vi "Format&SaveDataClean.vi"(0 "Data_Angle_deg":sgl[](array[numeric])=[490.08, 490.12, 490.16, 490.2], 1 "Data_PLInt_cts":i32[](array[numeric])=[1, 3, 2, 1], 3 "Data_FSMPos_V":dbl[][](array[numeric]), 4 "Data_CCD_px":dbl[][](array[numeric]), 5 "Measurement type":T3(ring)=enum."Contrast", 6 "L2Exc_deg":dbl[](array[numeric]), 7 "Suppl_2D":dbl[][](array[numeric]), 8 "L2Det_deg":dbl[](array[numeric]), 9 "Params Save":T2, 12 "Main 3D Data to write":dbl[][][](array[numeric])=[[[2.2, 4.4, 3.3, 5.5, 6.6]]], 13 "Suppl":dbl[](array[numeric]), 15 "Suppl_3D":dbl[][][](array[numeric])) -> (10 "WrittenDatasetName":string, 14 "Log File Out":string)   [LabVIEW 2019]
uses:
  TypeDefs/AcqMode.ctl
  <vilib>/UPVI/lvhdf5/dataset.llb/LVH5D Operation.ctl
  <vilib>/Utility/miscctls.llb/LVRectTypeDef.ctl
  <vilib>/UPVI/lvhdf5/attribute.llb/LVH5A Operation.ctl
  <vilib>/UPVI/lvhdf5/group.llb/H5G_obj_t.ctl
  <vilib>/UPVI/lvhdf5/identifier.llb/Not an HDF5 Refnum Constant.vi
  <vilib>/UPVI/lvhdf5/common.llb/To HDF5 Ref.vi
  <vilib>/UPVI/lvhdf5/group.llb/OpenCreateGroup (String).vi
  <vilib>/Utility/VariantDataType/GetClusterInfo.vi
  <vilib>/Utility/VariantDataType/GetTypeInfo.vi
  <vilib>/UPVI/lvhdf5/utility.llb/Select HDF5 Dialog.vi
  <vilib>/UPVI/lvhdf5/utility.llb/Select HDF5 Dialog (Object Only).vi
  <vilib>/UPVI/lvhdf5/dataset.llb/Simple H5Dwrite (Variant).vi
  <vilib>/UPVI/lvhdf5/attribute.llb/Write Multiple Attributes.vi
  <vilib>/UPVI/lvhdf5/dataset.llb/H5Dclose.vi
  <vilib>/UPVI/lvhdf5/dataset.llb/Write Dataset with Attributes.xnode
  <vilib>/UPVI/lvhdf5/library.llb/HDF5 Ref.ctl
  <vilib>/UPVI/lvhdf5/attribute.llb/Cluster to Attribute Array.xnode
  <vilib>/Utility/error.llb/Error Cluster From Error Code.vi
  <vilib>/UPVI/lvhdf5/dataset.llb/OpenCreateReplace Dataset by Element Type.vi
  <vilib>/UPVI/lvhdf5/dataspace.llb/H5Sselect_hyperslab.vi
  <vilib>/UPVI/lvhdf5/dataset.llb/H5Dwrite (Variant).vi
  <vilib>/UPVI/lvhdf5/dataset.llb/H5Dget_space.vi
  <vilib>/UPVI/lvhdf5/attribute.llb/private/LVH5AwriteWDTAttrs.vi
  <vilib>/UPVI/lvhdf5/dataspace.llb/H5Sclose.vi
  <vilib>/UPVI/lvhdf5/file.llb/LVH5F Operation.ctl
  <vilib>/UPVI/lvhdf5/utility.llb/Select HDF5 Dialog (File and Object).vi
  <vilib>/Utility/VariantDataType/VariantType.lvlib
panel:
  in  "ESource":enum16{"P", "CW", "SK"}(ring)
  in  "Acq Mode":T1=enum."Spectrum" caption="Acq mode"
  in  "Log File In":string
  out "File path":path=path "Cluster Attributes.hdf5"
  in  "DatasetName":string="test"
  in  "Main 2D Data to write":dbl[][](array[numeric])=[[2.2, 4.4, 3.3, 5.5, 6.6]]
  in  "Comment":string="This is a test"
  out "Date":string="2006-1-11"
  in  "T_K":dbl=5.0
  in  "EPow_uW":dbl=0.21
  in  "EWL_nm":dbl=450.0
  in  "Time_ms":dbl=500.0
  in  "Det_Mono1_EntSlit_mm":dbl=0.01
  in  "Det_Mono1_ExtSlit_mm":dbl=0.01
  in  "WL_nm":sgl[](array[numeric])=[490.08, 490.12, 490.16, 490.2]
  in  "MeasurementName":string
  in  "FileName":string="test"
  in  "Det_Mono1_CenterWL_nm":dbl=490.0
  out "Exists":bool
  out "Homonyms":string[](array[string])
  out "size(s)":i32
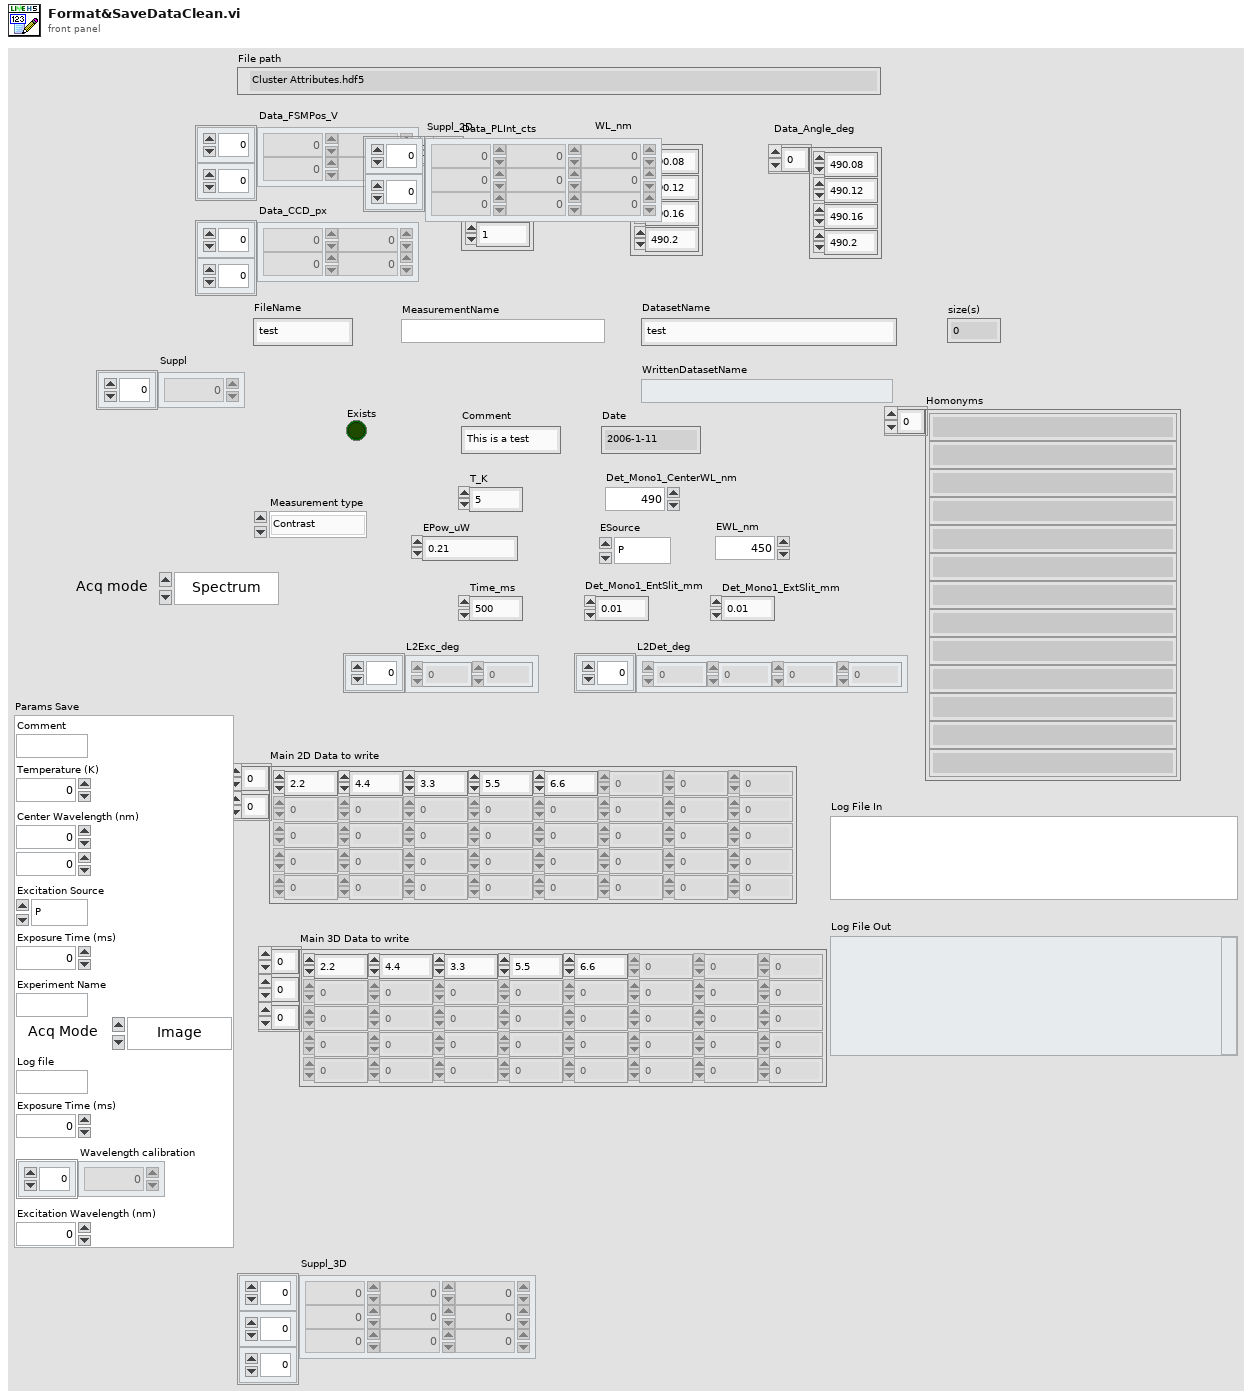
[diagram p1: front panel]
types:
  T1 = typedef "AcqMode.ctl" = enum16{"Image", "Spectrum", "APD 1", "APD 2", "APD 1+2"}
  T2 = cluster{"Comment":string, "Temperature (K)":dbl, "Center Wavelength (nm)":dbl, "Numeric":dbl, "Excitation Source":enum16{"P", "CW", "SK"}, "Exposure Time (ms)":dbl, "Experiment Name":string, "Acq Mode":T1, "Log file":string, "Exposure Time (ms)":dbl, "Wavelength calibration":dbl[], "Excitation Wavelength (nm)":dbl}
  T3 = enum16{"Time Trace", "Contrast", "XY Intensity Map", "Polarisation", "Spectrum", "Michelson"}
  T4 = typedef "LVH5D Operation.ctl" = enum16{"open", "replace", "create", "open or create", "create or replace", "create or replace with confirmation"}
  T5 = typedef "LVH5A Operation.ctl" = enum16{"open", "replace", "create", "open or create", "create or replace", "create or replace with confirmation"}
  T6 = typedef "LVRectTypeDef.ctl" = cluster{"Left":i16, "Top":i16, "Right":i16, "Bottom":i16}
  T7 = cluster{"Behavior":enum32{"Invalid", "Default", "Floating", "Floating/Auto-Hide", "Modal"}, "Position":T6, "Center":bool, "Title":string}
  T8 = typedef "LVH5F Operation.ctl" = enum16{"open", "open or create", "create or replace", "create or replace (with confirmation)", "create", "open (read only)"}
  T9 = typedef "H5G_obj_t.ctl" = i32
  T10 = cluster{"Object Types (any)":T9[], "Object Pattern":string}
  T11 = typedef "HDF5 Ref.ctl" = refnum<k1>
  T12 = cluster{"date/time string":string, "Comment":string, "T_K":dbl, "ESource":enum16{"P", "CW", "SK"}, "EWL_nm":dbl, "EPow_uW":dbl, "Time_ms":dbl, "WL_nm":sgl[], "Suppl":dbl[], "L2Exc_deg":dbl[], "L2Det_deg":dbl[]}
  T13 = cluster{"date/time string":string, "Comment":string, "T_K":dbl, "ESource":enum16{"P", "CW", "SK"}, "EWL_nm":dbl, "EPow_uW":dbl, "Time_ms":dbl, "WL_nm":sgl[], "Suppl_2D":dbl[][], "L2Exc_deg":dbl[], "L2Det_deg":dbl[]}
  T14 = cluster{"date/time string":string, "Comment":string, "T_K":dbl, "ESource":enum16{"P", "CW", "SK"}, "EWL_nm":dbl, "EPow_uW":dbl, "Time_ms":dbl, "WL_nm":sgl[], "Suppl_3D":dbl[][][], "L2Exc_deg":dbl[], "L2Det_deg":dbl[]}
  T15 = cluster{"date/time string":string, "Comment":string, "T_K":dbl, "ESource":enum16{"P", "CW", "SK"}, "EWL_nm":dbl, "EPow_uW":dbl, "Time_ms":dbl, "WL_nm":sgl[], "Suppl":dbl[], "L2Exc_deg":dbl[], "L2Det_deg":dbl[], "WL_nm":sgl[]}
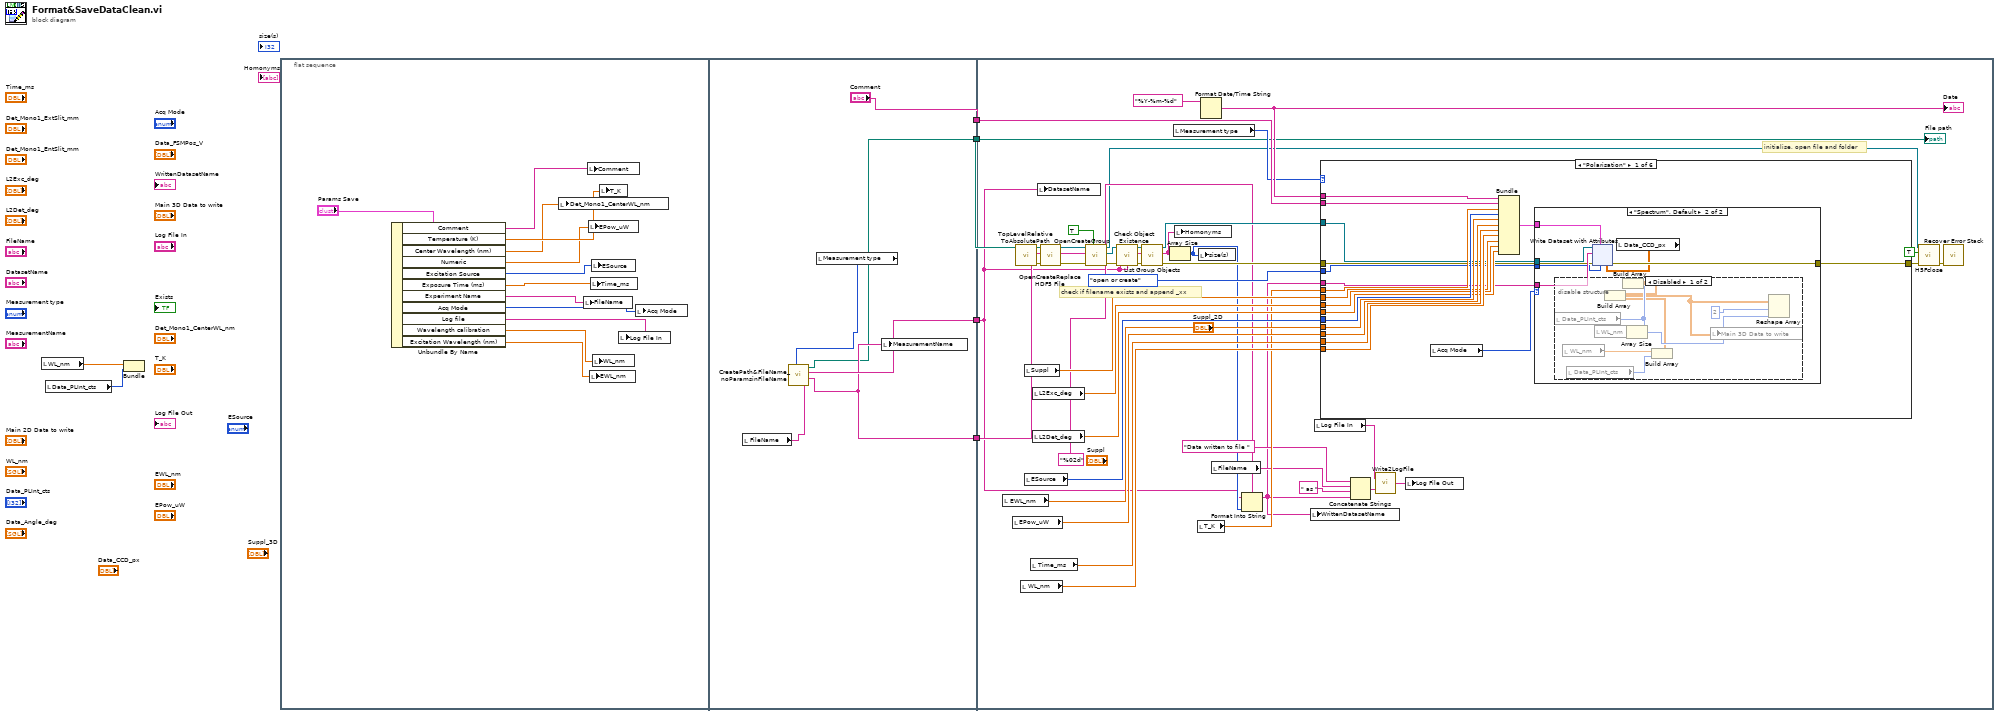
[diagram p0: block diagram]
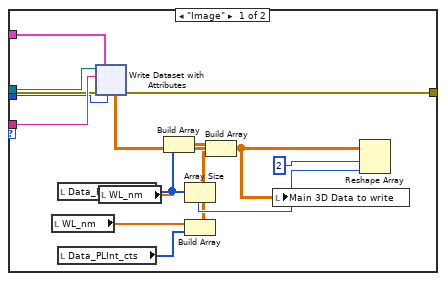
[diagram p2: hidden frame]
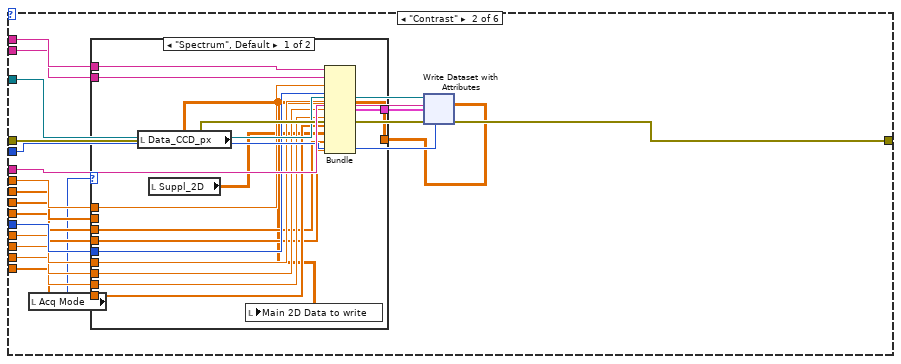
[diagram p4: hidden frame]
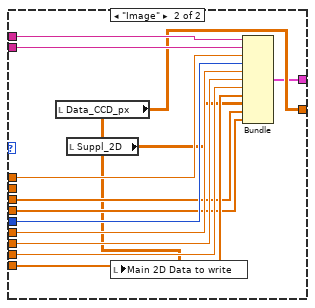
[diagram p5: hidden frame]
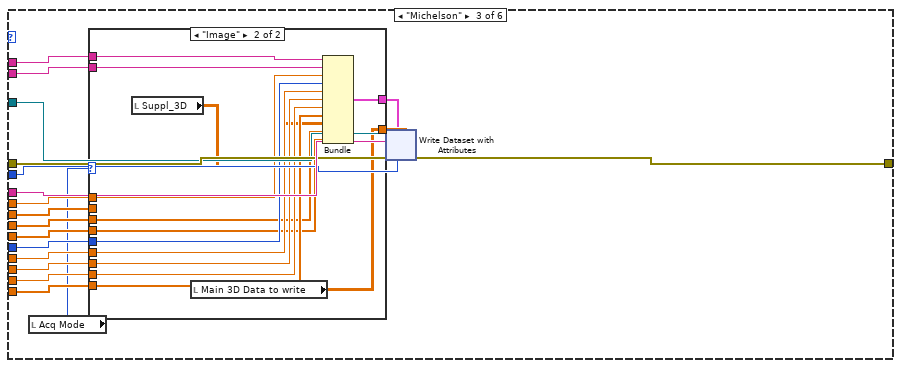
[diagram p6: hidden frame]
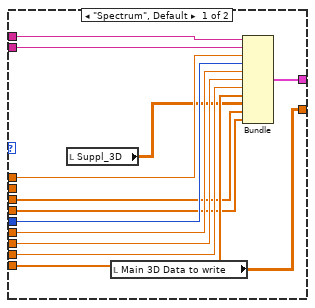
[diagram p7: hidden frame]
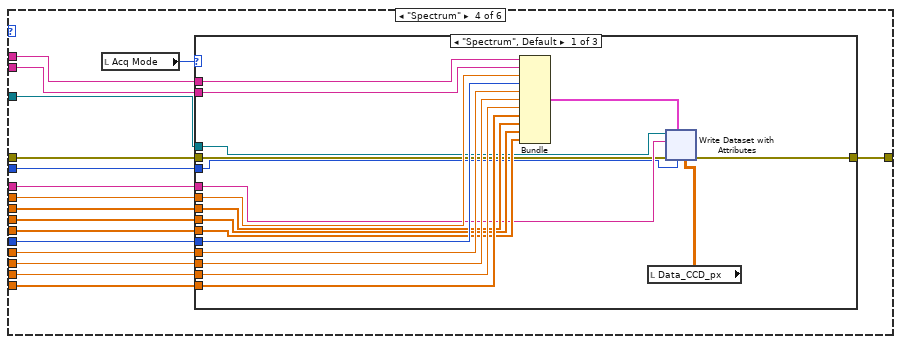
[diagram p8: hidden frame]
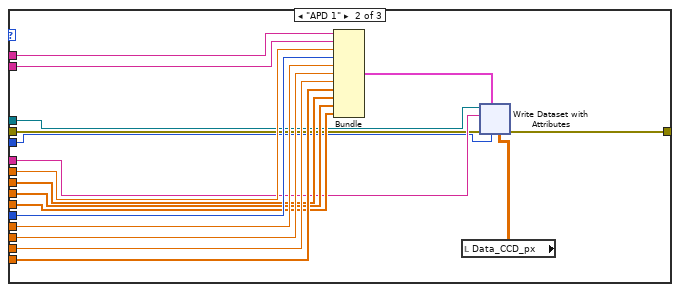
[diagram p9: hidden frame]
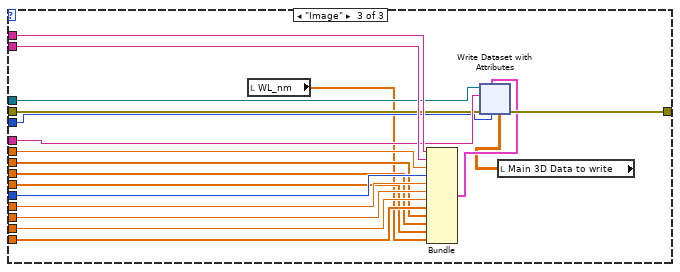
[diagram p10: hidden frame]
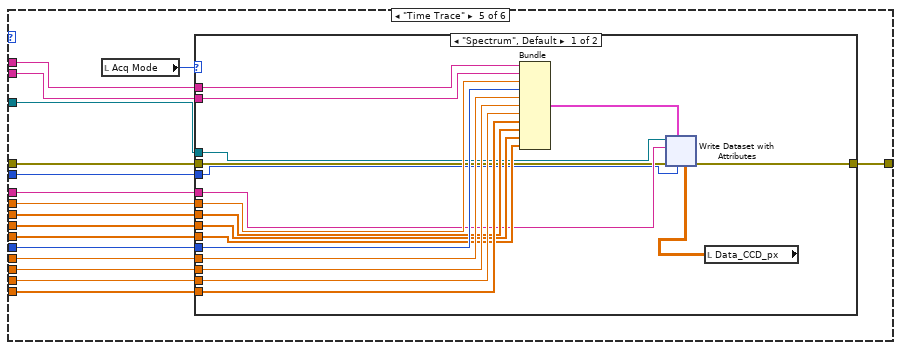
[diagram p11: hidden frame]
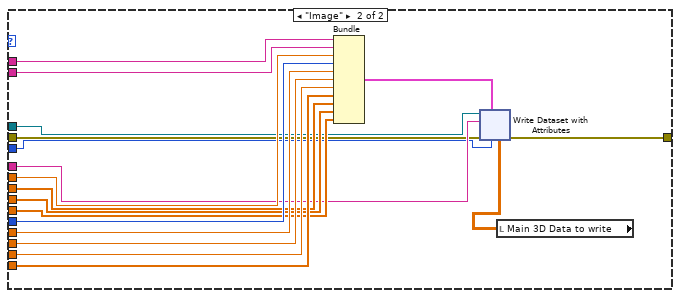
[diagram p12: hidden frame]
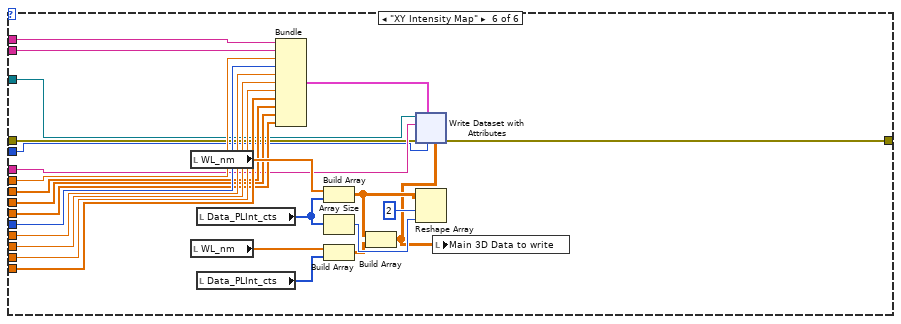
[diagram p13: hidden frame]
diagram:
  n1 = local read "WL_nm"() -> (w5:sgl[])
  n2 = local read "Data_PLInt_cts"() -> (w6:i32[])
  n3 = Bundle("WL_nm"=w5, "Data_PLInt_cts"=w6) -> ()  [unwired: 1 in, 1 out]
  n4 = flat-sequence {
    tunnel: ["Comment"] -> w4
    tunnel: [w22] -> w3
    tunnel: [w21] -> w2
    tunnel: [w20] -> w1
    tunnel: w4 -> [w53]
    tunnel: w3 -> [w25]
    tunnel: w2 -> [w43]
    tunnel: w1 -> [w36]
    frame #0 {
      n5 = Unbundle By Name("Params Save") -> ("Comment"=w17:string, "Temperature (K)"=w16:dbl, "Center Wavelength (nm)"=w14:dbl, "Numeric"=w15:dbl, "Excitation Source"=w13:enum16{"P", "CW", "SK"}, "Exposure Time (ms)"=w12:dbl, "Experiment Name"=w9:string, "Acq Mode"=w10:T1, "Log file"=w11:string, "Wavelength calibration"=w7:dbl[], "Excitation Wavelength (nm)"=w8:dbl)
      n6 = local write "Det_Mono1_CenterWL_nm"(w14) -> ()
      n7 = local write "FileName"(w9) -> ()
      n8 = local write "Comment"(w17) -> ()
      n9 = local write "EPow_uW"(w15) -> ()
      n10 = local write "EWL_nm"(w8) -> ()
      n11 = local write "Time_ms"(w12) -> ()
      n12 = local write "ESource"(w13) -> ()
      n13 = local write "WL_nm"(w7) -> ()
      n14 = local write "T_K"(w16) -> ()
      n15 = local write "Log File In"(w11) -> ()
      n16 = local write "Acq Mode"(w10) -> ()
    }
    frame #1 {
      n17 = local read "FileName"() -> (w19:string)
      n18 = local read "Measurement type"() -> (w23:T3)
      n19 = call "CreatePath&FileName_noParamsinFileName.vi"("FileName"=w19, "Measurement type"=w23) -> ("MeasurementGroupName"=w21:string, "DatasetName"=w22:string, "File path"=w20:path)  [unwired: 4 in]
      n20 = local write "MeasurementName"(w21) -> ()
    }
    frame #2 {
      # "initialise, open file and folder"
      # "check if filename exists and append _xx"
      n21 = local read "EWL_nm"() -> (w56:dbl)
      n22 = local read "EPow_uW"() -> (w57:dbl)
      n23 = call "TopLevelRelativeToAbsolutePath.vi"("Path Relative to Top Level VI"=w36) -> ("error out"=w34:errorcluster, "Absolute path"=w33:path)  [unwired: 9 in]
      n24 = local read "WL_nm"() -> (w59:sgl[])
      n25 = local read "Suppl"() -> (w60:dbl[])
      n26 = local read "ESource"() -> (w55:enum16{"P", "CW", "SK"})
      n27 = local read "Time_ms"() -> (w58:dbl)
      n28 = local read "L2Exc_deg"() -> (w61:dbl[])
      n29 = local read "L2Det_deg"() -> (w62:dbl[])
      n30 = local write "DatasetName"(w25) -> ()
      n31 = call <vilib>:"OpenCreateReplace HDF5 File.vi"("error in (no error)"=w34, "path"=w33) -> ("error out"=w38:errorcluster, "HDF5 Ref out"=w37:T11)  [unwired: 6 in]
      n32 = call-poly <vilib>:"OpenCreateGroup.vi"("Create if not found (F)"=TRUE, "error in (no error)"=w38, "Group"=w43, "HDF5 Ref"=w37) -> ("error out"=w46:errorcluster, "HDF5 Group Ref"=w45:T11, "HDF5 Ref out"=w41:T11)  [unwired: 5 in]
      n33 = call <vilib>:"Check Object Existence.vi"("error in (no error)"=w46, "name"=w25, "HDF5 Ref"=w45) -> ("error out"=w47:errorcluster, "HDF5 Ref out"=w48:T11)  [unwired: 4 in, 1 out]
      n34 = call <vilib>:"List Group Objects.vi"("error in (no error)"=w47, "pattern"=w25, "HDF5 Loc Ref"=w48) -> ("error out"=w63:errorcluster, "Object Names"=w49:string[], "HDF5 Loc Ref out"=w65:T11)  [unwired: 3 in, 1 out]
      n35 = Array Size(array=w49) -> (size(s)=w50:i32)
      n36 = local read "Measurement type"() -> (w42:T3)
      n37 = local write "Homonyms"(w49) -> ()
      n38 = local read "T_K"() -> (w54:dbl)
      n39 = local write "size(s)"(w50) -> ()
      n40 = Format Date/Time String(time format string (%c)="%Y-%m-%d") -> (date/time string=w52:string)  [unwired: 2 in]
      "Date" <- w52
      n41 = local read "FileName"() -> (w31:string)
      n42 = Format Into String(format string="%02d", initial string=w25, w50) -> (resulting string=w29:string)  [unwired: 1 in, 1 out]
      n43 = local write "WrittenDatasetName"(w29) -> ()
      n44 = local read "Log File In"() -> (w28:string)
      n45 = case shown="\"Polarisation\"" w42 {
        tunnel: w52 -> [w84 w762 w1121 w1478 w2494 w3180]
        tunnel: w53 -> [w83 w761 w1120 w1477 w2493 w3179]
        tunnel: w54 -> [w82 w760 w1119 w1476 w2492 w3178]
        tunnel: w55 -> [w81 w759 w1118 w1475 w2491 w3177]
        tunnel: w56 -> [w80 w758 w1117 w1474 w2490 w3176]
        tunnel: w57 -> [w79 w757 w1116 w1473 w2489 w3175]
        tunnel: w58 -> [w78 w756 w1115 w1472 w2488 w3174]
        tunnel: w59 -> [w77 w755 w1114 w1471 w2487 w3173]
        tunnel: w60 -> [w76 w754 w1113 w1470 w2486 w3172]
        tunnel: w61 -> [w75 w753 w1112 w1469 w2485 w3171]
        tunnel: w62 -> [w74 w752 w1111 w1468 w2484 w3170]
        tunnel: w29 -> [w73 w751 w1110 w1467 w2483 w3169]
        tunnel: w63 -> [w72 w750 w1109 w1466 w2482 w3168]
        tunnel: LVH5D_Operation."open or create" ("operation (open or create)") -> [w71 w749 w1108 w1465 w2481 w3167]
        tunnel: w65 -> [w70 w748 w1107 w1464 w2480 w3166]
        tunnel: [w69 w747 w1106 w1463 w2479 w3165] -> w66
        frame "Polarisation" {
          n46 = local read "Acq Mode"() -> (w68:T1)
          n47 = Bundle("date/time string"=w84, "Comment"=w83, "T_K"=w82, "ESource"=w81, "EWL_nm"=w80, "EPow_uW"=w79, "Time_ms"=w78, "WL_nm"=w77, "Suppl"=w76, "L2Exc_deg"=w75, "L2Det_deg"=w74) -> (w67:T12)  [unwired: 1 in]
          n48 = case shown="\"Spectrum\", Default" w68 {
            tunnel: w73 -> [w95 w420]
            tunnel: w72 -> [w94 w419]
            tunnel: w71 -> [w93 w418]
            tunnel: w70 -> [w92 w417]
            tunnel: [w91 w416] -> w69
            tunnel: w67 -> [w85 w415]
            frame "Image" {
              n49 = local read "WL_nm"() -> (w90:sgl[])
              n50 = local read "Data_PLInt_cts"() -> (w97:i32[])
              n51 = local read "Data_PLInt_cts"() -> (w89:i32[])
              n52 = local read "WL_nm"() -> (w96:sgl[])
              n53 = Build Array(w96, w97) -> (w87:sgl[][])
              n54 = Array Size(array=w97) -> (size(s)=w98:i32)
              n55 = Build Array(w90, w89) -> (w88:sgl[][])
              n56 = Build Array(w87, w88) -> (w86:sgl[][][])
              n57 = xnode "Write Dataset with Attributes"("Dataset Path"=w95, "error in (no error)"=w94, "operation (open or create)"=w93, "HDF5 Path or Ref"=w92, "Attribute Value(s)"=w85, "Data"=w86) -> ("error out"=w91:errorcluster)  [unwired: 2 in, 2 out]
              n58 = local write "Main 3D Data to write"(w86) -> ()
              n59 = Reshape Array(w86, 2 ("dimension size"), w98) -> ()  [unwired: 1 out]
            }
            frame "Spectrum", Default {
              n60 = disable-structure shown="Disabled" {
                frame Disabled {
                  n61 = local read "Data_PLInt_cts"() -> (w427:i32[])
                  n62 = local read "WL_nm"() -> (w425:sgl[])
                  n63 = local read "Data_PLInt_cts"() -> (w424:i32[])
                  n64 = local read "WL_nm"() -> (w426:sgl[])
                  n65 = Build Array(w426, w427) -> (w422:sgl[][])
                  n66 = Array Size(array=w427) -> (size(s)=w428:i32)
                  n67 = Build Array(w425, w424) -> (w423:sgl[][])
                  n68 = Build Array(w422, w423) -> (w421:sgl[][][])
                  n69 = local write "Main 3D Data to write"(w421) -> ()
                  n70 = Reshape Array(w421, 2 ("dimension size"), w428) -> ()  [unwired: 1 out]
                }
                frame Enabled {
                }
              }
              n71 = local read "Data_CCD_px"() -> (w414:dbl[][])
              n72 = xnode "Write Dataset with Attributes"("Dataset Path"=w420, "error in (no error)"=w419, "operation (open or create)"=w418, "HDF5 Path or Ref"=w417, "Attribute Value(s)"=w415, "Data"=w414) -> ("error out"=w416:errorcluster)  [unwired: 2 in, 2 out]
            }
          }
        }
        frame "Contrast" {
          n73 = local read "Acq Mode"() -> (w745:T1)
          n74 = case shown="\"Spectrum\", Default" w745 {
            tunnel: w762 -> [w775 w788]
            tunnel: w761 -> [w774 w787]
            tunnel: w760 -> [w773 w786]
            tunnel: w759 -> [w772 w785]
            tunnel: w758 -> [w771 w784]
            tunnel: w757 -> [w770 w783]
            tunnel: w756 -> [w769 w782]
            tunnel: w755 -> [w768 w781]
            tunnel: w754 -> [_ _]
            tunnel: w753 -> [w767 w780]
            tunnel: w752 -> [w766 w779]
            tunnel: [w765 w778] -> w746
            tunnel: [w763 w777] -> w744
            frame "Spectrum", Default {
              n75 = local read "Data_CCD_px"() -> (w765:dbl[][])
              n76 = local read "Suppl_2D"() -> (w764:dbl[][])
              n77 = local write "Main 2D Data to write"(w765) -> ()
              n78 = Bundle("date/time string"=w775, "Comment"=w774, "T_K"=w773, "ESource"=w772, "EWL_nm"=w771, "EPow_uW"=w770, "Time_ms"=w769, "WL_nm"=w768, "Suppl_2D"=w764, "L2Exc_deg"=w767, "L2Det_deg"=w766) -> (w763:T13)  [unwired: 1 in]
            }
            frame "Image" {
              n79 = local read "Data_CCD_px"() -> (w778:dbl[][])
              n80 = local read "Suppl_2D"() -> (w776:dbl[][])
              n81 = local write "Main 2D Data to write"(w778) -> ()
              n82 = Bundle("date/time string"=w788, "Comment"=w787, "T_K"=w786, "ESource"=w785, "EWL_nm"=w784, "EPow_uW"=w783, "Time_ms"=w782, "WL_nm"=w781, "Suppl_2D"=w776, "L2Exc_deg"=w780, "L2Det_deg"=w779) -> (w777:T13)  [unwired: 1 in]
            }
          }
          n83 = xnode "Write Dataset with Attributes"("Dataset Path"=w751, "error in (no error)"=w750, "operation (open or create)"=w749, "HDF5 Path or Ref"=w748, "Attribute Value(s)"=w744, "Data"=w746) -> ("error out"=w747:errorcluster)  [unwired: 2 in, 2 out]
        }
        frame "Michelson" {
          n84 = local read "Acq Mode"() -> (w1104:T1)
          n85 = case shown="\"Image\"" w1104 {
            tunnel: w1121 -> [w1134 w1147]
            tunnel: w1120 -> [w1133 w1146]
            tunnel: w1119 -> [w1132 w1145]
            tunnel: w1118 -> [w1131 w1144]
            tunnel: w1117 -> [w1130 w1143]
            tunnel: w1116 -> [w1129 w1142]
            tunnel: w1115 -> [w1128 w1141]
            tunnel: w1114 -> [w1127 w1140]
            tunnel: w1113 -> [_ _]
            tunnel: w1112 -> [w1126 w1139]
            tunnel: w1111 -> [w1125 w1138]
            tunnel: [w1123 w1137] -> w1105
            tunnel: [w1124 w1135] -> w1103
            frame "Spectrum", Default {
              n86 = local read "Suppl_3D"() -> (w1122:dbl[][][])
              n87 = local read "Main 3D Data to write"() -> (w1123:dbl[][][])
              n88 = Bundle("date/time string"=w1134, "Comment"=w1133, "T_K"=w1132, "ESource"=w1131, "EWL_nm"=w1130, "EPow_uW"=w1129, "Time_ms"=w1128, "WL_nm"=w1127, "Suppl_3D"=w1122, "L2Exc_deg"=w1126, "L2Det_deg"=w1125) -> (w1124:T14)  [unwired: 1 in]
            }
            frame "Image" {
              n89 = local read "Suppl_3D"() -> (w1136:dbl[][][])
              n90 = local read "Main 3D Data to write"() -> (w1137:dbl[][][])
              n91 = Bundle("date/time string"=w1147, "Comment"=w1146, "T_K"=w1145, "ESource"=w1144, "EWL_nm"=w1143, "EPow_uW"=w1142, "Time_ms"=w1141, "WL_nm"=w1140, "Suppl_3D"=w1136, "L2Exc_deg"=w1139, "L2Det_deg"=w1138) -> (w1135:T14)  [unwired: 1 in]
            }
          }
          n92 = xnode "Write Dataset with Attributes"("Dataset Path"=w1110, "error in (no error)"=w1109, "operation (open or create)"=w1108, "HDF5 Path or Ref"=w1107, "Attribute Value(s)"=w1103, "Data"=w1105) -> ("error out"=w1106:errorcluster)  [unwired: 2 in, 2 out]
        }
        frame "Spectrum" {
          n93 = local read "Acq Mode"() -> (w1462:T1)
          n94 = case shown="\"Spectrum\", Default" w1462 {
            tunnel: w1478 -> [w1496 w1828 w2161]
            tunnel: w1477 -> [w1495 w1827 w2160]
            tunnel: w1476 -> [w1494 w1826 w2159]
            tunnel: w1475 -> [w1493 w1825 w2158]
            tunnel: w1474 -> [w1492 w1824 w2157]
            tunnel: w1473 -> [w1491 w1823 w2156]
            tunnel: w1472 -> [w1490 w1822 w2155]
            tunnel: w1471 -> [w1489 w1821 w2154]
            tunnel: w1470 -> [w1488 w1820 w2153]
            tunnel: w1469 -> [w1487 w1819 w2152]
            tunnel: w1468 -> [w1486 w1818 w2151]
            tunnel: w1467 -> [w1485 w1817 w2150]
            tunnel: w1466 -> [w1484 w1816 w2149]
            tunnel: w1465 -> [w1483 w1815 w2148]
            tunnel: w1464 -> [w1482 w1814 w2147]
            tunnel: [w1481 w1813 w2146] -> w1463
            frame "Spectrum", Default {
              n95 = Bundle("date/time string"=w1496, "Comment"=w1495, "T_K"=w1494, "ESource"=w1493, "EWL_nm"=w1492, "EPow_uW"=w1491, "Time_ms"=w1490, "WL_nm"=w1489, "Suppl"=w1488, "L2Exc_deg"=w1487, "L2Det_deg"=w1486) -> (w1480:T12)  [unwired: 1 in]
              n96 = local read "Data_CCD_px"() -> (w1479:dbl[][])
              n97 = xnode "Write Dataset with Attributes"("Dataset Path"=w1485, "error in (no error)"=w1484, "operation (open or create)"=w1483, "HDF5 Path or Ref"=w1482, "Attribute Value(s)"=w1480, "Data"=w1479) -> ("error out"=w1481:errorcluster)  [unwired: 2 in, 2 out]
            }
            frame "APD 1" {
              n98 = Bundle("date/time string"=w1828, "Comment"=w1827, "T_K"=w1826, "ESource"=w1825, "EWL_nm"=w1824, "EPow_uW"=w1823, "Time_ms"=w1822, "WL_nm"=w1821, "Suppl"=w1820, "L2Exc_deg"=w1819, "L2Det_deg"=w1818) -> (w1812:T12)  [unwired: 1 in]
              n99 = local read "Data_CCD_px"() -> (w1811:dbl[][])
              n100 = xnode "Write Dataset with Attributes"("Dataset Path"=w1817, "error in (no error)"=w1816, "operation (open or create)"=w1815, "HDF5 Path or Ref"=w1814, "Attribute Value(s)"=w1812, "Data"=w1811) -> ("error out"=w1813:errorcluster)  [unwired: 2 in, 2 out]
            }
            frame "Image" {
              n101 = local read "WL_nm"() -> (w2145:sgl[])
              n102 = Bundle("date/time string"=w2161, "Comment"=w2160, "T_K"=w2159, "ESource"=w2158, "EWL_nm"=w2157, "EPow_uW"=w2156, "Time_ms"=w2155, "WL_nm"=w2154, "Suppl"=w2153, "L2Exc_deg"=w2152, "L2Det_deg"=w2151, "WL_nm"=w2145) -> (w2144:T15)  [unwired: 1 in]
              n103 = local read "Main 3D Data to write"() -> (w2143:dbl[][][])
              n104 = xnode "Write Dataset with Attributes"("Dataset Path"=w2150, "error in (no error)"=w2149, "operation (open or create)"=w2148, "HDF5 Path or Ref"=w2147, "Attribute Value(s)"=w2144, "Data"=w2143) -> ("error out"=w2146:errorcluster)  [unwired: 2 in, 2 out]
            }
          }
        }
        frame "Time Trace" {
          n105 = local read "Acq Mode"() -> (w2478:T1)
          n106 = case shown="\"Spectrum\", Default" w2478 {
            tunnel: w2494 -> [w2512 w2844]
            tunnel: w2493 -> [w2511 w2843]
            tunnel: w2492 -> [w2510 w2842]
            tunnel: w2491 -> [w2509 w2841]
            tunnel: w2490 -> [w2508 w2840]
            tunnel: w2489 -> [w2507 w2839]
            tunnel: w2488 -> [w2506 w2838]
            tunnel: w2487 -> [w2505 w2837]
            tunnel: w2486 -> [w2504 w2836]
            tunnel: w2485 -> [w2503 w2835]
            tunnel: w2484 -> [w2502 w2834]
            tunnel: w2483 -> [w2501 w2833]
            tunnel: w2482 -> [w2500 w2832]
            tunnel: w2481 -> [w2499 w2831]
            tunnel: w2480 -> [w2498 w2830]
            tunnel: [w2497 w2829] -> w2479
            frame "Spectrum", Default {
              n107 = Bundle("date/time string"=w2512, "Comment"=w2511, "T_K"=w2510, "ESource"=w2509, "EWL_nm"=w2508, "EPow_uW"=w2507, "Time_ms"=w2506, "WL_nm"=w2505, "Suppl"=w2504, "L2Exc_deg"=w2503, "L2Det_deg"=w2502) -> (w2496:T12)  [unwired: 1 in]
              n108 = local read "Data_CCD_px"() -> (w2495:dbl[][])
              n109 = xnode "Write Dataset with Attributes"("Dataset Path"=w2501, "error in (no error)"=w2500, "operation (open or create)"=w2499, "HDF5 Path or Ref"=w2498, "Attribute Value(s)"=w2496, "Data"=w2495) -> ("error out"=w2497:errorcluster)  [unwired: 2 in, 2 out]
            }
            frame "Image" {
              n110 = Bundle("date/time string"=w2844, "Comment"=w2843, "T_K"=w2842, "ESource"=w2841, "EWL_nm"=w2840, "EPow_uW"=w2839, "Time_ms"=w2838, "WL_nm"=w2837, "Suppl"=w2836, "L2Exc_deg"=w2835, "L2Det_deg"=w2834) -> (w2828:T12)  [unwired: 1 in]
              n111 = local read "Main 3D Data to write"() -> (w2827:dbl[][][])
              n112 = xnode "Write Dataset with Attributes"("Dataset Path"=w2833, "error in (no error)"=w2832, "operation (open or create)"=w2831, "HDF5 Path or Ref"=w2830, "Attribute Value(s)"=w2828, "Data"=w2827) -> ("error out"=w2829:errorcluster)  [unwired: 2 in, 2 out]
            }
          }
        }
        frame "XY Intensity Map" {
          n113 = local read "WL_nm"() -> (w3181:sgl[])
          n114 = local read "WL_nm"() -> (w3164:sgl[])
          n115 = local read "Data_PLInt_cts"() -> (w3182:i32[])
          n116 = local read "Data_PLInt_cts"() -> (w3160:i32[])
          n117 = Bundle("date/time string"=w3180, "Comment"=w3179, "T_K"=w3178, "ESource"=w3177, "EWL_nm"=w3176, "EPow_uW"=w3175, "Time_ms"=w3174, "WL_nm"=w3173, "Suppl"=w3172, "L2Exc_deg"=w3171, "L2Det_deg"=w3170) -> (w3159:T12)  [unwired: 1 in]
          n118 = Build Array(w3181, w3182) -> (w3162:sgl[][])
          n119 = Array Size(array=w3182) -> (size(s)=w3183:i32)
          n120 = Build Array(w3164, w3160) -> (w3163:sgl[][])
          n121 = Build Array(w3162, w3163) -> (w3161:sgl[][][])
          n122 = xnode "Write Dataset with Attributes"("Dataset Path"=w3169, "error in (no error)"=w3168, "operation (open or create)"=w3167, "HDF5 Path or Ref"=w3166, "Attribute Value(s)"=w3159, "Data"=w3161) -> ("error out"=w3165:errorcluster)  [unwired: 2 in, 2 out]
          n123 = Reshape Array(w3162, 2 ("dimension size"), w3183) -> ()  [unwired: 1 out]
          n124 = local write "Main 3D Data to write"(w3161) -> ()
        }
      }
      n125 = Concatenate Strings("Data written to file ", w31, " as ", w29) -> (w27:string)
      n126 = call "Write2LogFile.vi"("Add to log file"=w27, "Log file before"=w28) -> ("Log file after"=w26:string)
      n127 = local write "Log File Out"(w26) -> ()
      n128 = call <vilib>:"H5Fclose.vi"("error in (no error)"=w66, "Close All Open Objects (T)"=TRUE, "HDF5 Ref"=w41) -> ("error out"=w39:errorcluster)  [unwired: 6 in]
      n129 = call <vilib>:"Recover Error Stack.vi"("error in (no error)"=w39) -> ()  [unwired: 5 in, 4 out]
      "File path" <- w36
    }
  }
